vi "Constructor.vi"(9 "Y Range":dbl[](array[numeric]), 10 "X Range":dbl[](array[numeric]), 11 "Sample Rate":i32) -> (3 "Exponential Fit out":refnum<class "Exponential Fit.lvclass">)   [LabVIEW 2016, in "Exponential Fit.lvclass"]
uses:
  Exponential Fit.lvclass
  Exponential Fit.lvclass/Exponential Fit.ctl
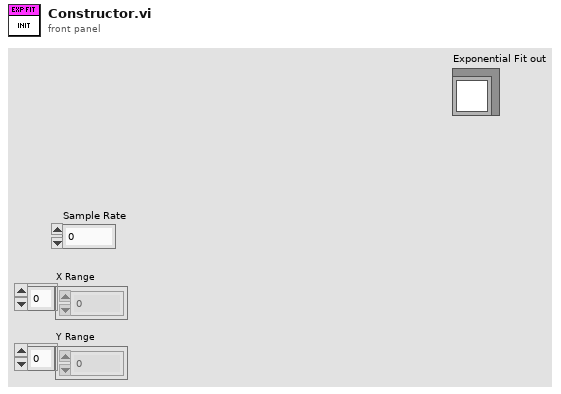
[diagram p1: front panel]
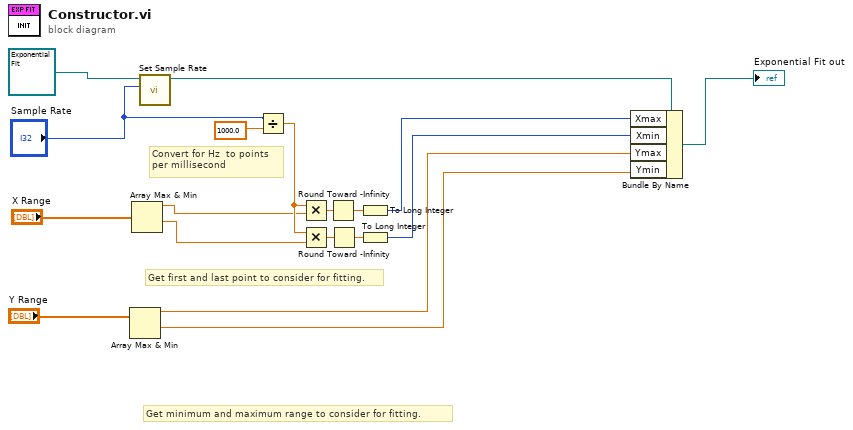
[diagram p0: block diagram]
diagram:
  # "Get minimum and maximum range to consider for fitting."
  # "Get first and last point to consider for fitting."
  # "Convert for Hz  to points\nper millisecond"
  n1 = Array Max & Min(array="Y Range") -> (max value=w2:dbl, min value=w1:dbl)  [unwired: 2 out]
  n2 = Array Max & Min(array="X Range") -> (max value=w8:dbl, min value=w7:dbl)  [unwired: 2 out]
  n3 = call-dynamic "Set Sample Rate.vi"("Sample Rate"="Sample Rate", "Abstract Fit in"=refnum<class "Exponential Fit.lvclass"> refnum ("Exponential Fit.lvclass")) -> ("Abstract Fit out"=w15:refnum<class "Exponential Fit.lvclass">)  [unwired: 8 in, 1 out]
  n4 = Divide(x="Sample Rate", y=1000.0) -> (x/y=w9:dbl)
  n5 = Multiply(x=w9, y=w8) -> (x*y=w12:dbl)
  n6 = Multiply(x=w9, y=w7) -> (x*y=w13:dbl)
  n7 = Round Toward -Infinity(1:w12) -> (0:w11:dbl)
  n8 = Round Toward -Infinity(1:w13) -> (0:w10:dbl)
  n9 = To Long Integer(number=w11) -> (32bit integer=w6:i32)
  n10 = To Long Integer(number=w10) -> (32bit integer=w5:i32)
  n11 = Bundle By Name(cluster=w15, "Xmax"=w6, "Xmin"=w5, "Ymax"=w2, "Ymin"=w1) -> (→"Exponential Fit out":refnum<class "Exponential Fit.lvclass">)
